vi "AlliGator Save Decay Fit Parameter Map Image.vi"(6 "Dialog?":bool, 8 "error in (no error)":errorcluster, 9 "Fit Parameter":T2, 10 "Image Control Refnum":T1, 11 "IV DVR":refnum<data-value>) -> (0 "error out":errorcluster, 2 "Message":string, 3 "IV DVR":refnum<data-value>)   [LabVIEW 2021, in "AlliGator Decay Fit Parameter Map.lvlib"]
uses:
  AlliGator Decay Fit Parameter Map.lvlib
  Image/Image.lvlib
  Files/AlliGator Files.lvlib
  Internal Variables/AlliGator Internal Variables.lvlib
  Phasor/Phasor Reference Series.ctl
  Phasor/Phasor.lvlib
  Phasor/Calibration Phasor (m, phi).ctl
  Phasor/Phasor (g, s).ctl
  <vilib>/vision/Image Controls.llb/IMAQ Image.ctl
  Image/Named ROI Description.ctl
  Decay Analysis/Decay Preprocessing/AlliGator Baseline Subtraction Method.ctl
  Decay Analysis/Decay Preprocessing/AlliGator Decay Preprocessing.lvlib
  Decay Analysis/Decay Preprocessing/AlliGator Decay Background Subtraction Info.ctl
  Graphs/XY Graph/XY Graph Plot Shift Method.ctl
  Graphs/XY Graph/XY Graph Add-Ons.lvlib
  Graphs/XY Graph/XY Graph Plot Shift Parameters.ctl
  Decay Analysis/Decay Preprocessing/AlliGator Decay Extrapolation Parameters.ctl
  Phasor Graph/AlliGator Decay Metadata v3.ctl
  Phasor Graph/AlliGator Phasor Graph.lvlib
  Phasor/Phasor Standard Deviation Options.ctl
  Phasor Graph/AlliGator Raw Phasor Plot Data v4.ctl
  Files/AlliGator Data Series Type.ctl
  Internal Variables/AlliGator Gate Image Set.ctl
  Phasor/Phasor Calibration Map v2.ctl
  Files/AlliGator FLI Dataset Type.ctl
  Phasor/Phasor Harmonic Data.ctl
  Phasor Plot/AlliGator Phasor Multi-Harmonic Data.ctl
  Phasor Plot/AlliGator Phasor Plot.lvlib
  Source Image/AlliGator Displayed Image.ctl
  Source Image/AlliGator Source Image.lvlib
  Fits/IRF(X)PSED/Decay Fit Parameters & Derived Quantities List v2.ctl
  Fits/Fits.lvlib
  Fits/IRF(X)PSED/Decay Fit Parameters In List.ctl
  Decay Analysis/Decay Fit/AlliGator Decay Fit Parameter Constraints 2.ctl
  Decay Analysis/Decay Fit/AlliGator Decay Fit.lvlib
  Fits/Decay Convolution/Decay Model.ctl
  Fits/Residual Type.ctl
  Fits/IRF(X)PSED/Fit Weights Type.ctl
  Fits/Non-linear Fitting Method v2.ctl
  Fits/Fit Calculation Method.ctl
  Fits/Non-linear Fitting Algorithm.ctl
  Fits/IRF(X)PSED/Decay Fit Options v2.ctl
  Fits/IRF(X)PSED/MLE Baseline Offset Type.ctl
  AlliGator Decay Fit Options & Parameters v2.ctl
  Settings/AlliGator Gate Arithmetic.ctl
  Settings/AlliGator Settings.lvlib
  Dual-Channel Datasets/AlliGator Dataset Channel.ctl
  Dual-Channel Datasets/AlliGator Dual-Channel Datasets.lvlib
  Decay Analysis/Decay Preprocessing/AlliGator Decay Preprocessing Parameters.ctl
  AlliGator Parameter Maps Data.ctl
  Internal Variables/AlliGator Internal Variables v2.ctl
  Image/Image Control Refnum.ctl
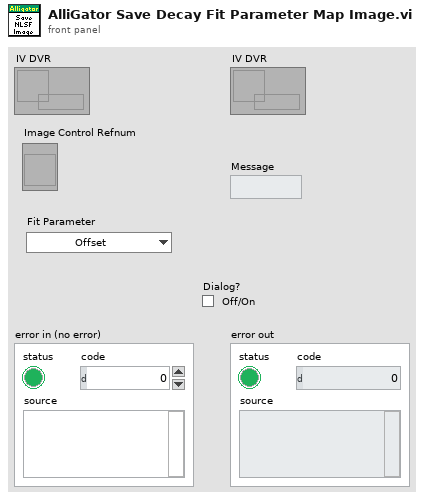
[diagram p1: front panel]
types:
  T1 = typedef "Image.lvlib/Image Control Refnum.ctl" = refnum<vi>
  T2 = typedef "Fits.lvlib/Decay Fit Parameters & Derived Quantities List v2.ctl" = enum16{"Offset", "Baseline", "A_1", "tau_1", "A_2", "tau_2", "<tau>_a", "f1_a", "f2_a", "<tau>_i", "f1_i", "f2_i", "-", "R^2", "Chi^2"}
  T3 = typedef "Image.lvlib/Image Save File Format.ctl" = enum16{"PNG", "JPEG", "BMP"}
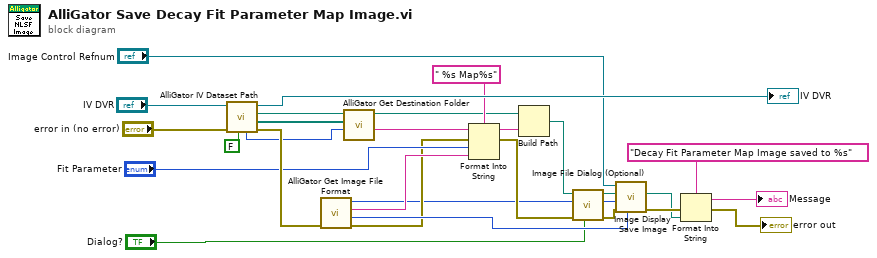
[diagram p0: block diagram]
diagram:
  n1 = call "AlliGator IV Dataset Path.vi"("Get (F)/ Set (T)"=FALSE, "error in (no error)"="error in (no error)", "AlliGator IV DVR in"="IV DVR") -> ("error out"=w25:errorcluster, "[Time-Series Path]"=w20:path[], "Single Data Point Path"=w19:path, "AlliGator IV DVR out"=→"IV DVR":refnum<data-value>, "Current Dataset"=w21:i32)  [unwired: 4 in]
  n2 = call "AlliGator Get Image File Format.vi"("Error In"=w25) -> ("error out"=w10:errorcluster, "Transparent Mask Color"=w28:u32, "File Extension (.xxx)"=w13:string, "Image File Format"=w5:T3)  [unwired: 7 in]
  n3 = call "AlliGator Get Destination Folder.vi"("Current Data Set (-1: single)"=w21, "Time-Series Paths"=w20, "Single Data Point Path"=w19) -> ("Data Point Name"=w8:string, "Destination Folder path"=w2:path)  [unwired: 6 in, 1 out]
  n4 = Format Into String(format string=" %s Map%s", initial string=w8, error in=w10, "Fit Parameter", w13) -> (resulting string=w11:string, error out=w12:errorcluster)
  n5 = Build Path(base path=w2, name or relative path=w11) -> (appended path=w3:path)
  n6 = call "Image File Dialog (Optional).vi"("Dialog?"="Dialog?", "Error In"=w12, "Image File Format in"=w5, "Default file path in"=w3) -> ("Error Out"=w18:errorcluster, "Image File Format out"=w6:T3, "file path out"=w4:path)  [unwired: 5 in]
  n7 = call "Image Display Save Image.vi"("Mask Color (Transparent)"=w28, "error in (no error)"=w18, "Saved Image File Format"=w6, "File Path in"=w4, "Display Image Control Refnum"="Image Control Refnum") -> ("Error Out"=w17:errorcluster, "File Path out"=w16:path)  [unwired: 5 in]
  n8 = Format Into String(format string="Decay Fit Parameter Map Image saved to %s", error in=w17, w16) -> (resulting string=→"Message":string, error out=→"error out":errorcluster)  [unwired: 1 in]
